vi "Excel_Insert_Table.vi"(0 "worksheet":refnum<k7>, 1 "font":T1 {"font size" format="%0.2f"; "strike through" items=["Unchanged", "Yes", "No"]; "underline" items=["Unchanged", "Yes", "No"]; "italic" items=["Unchanged", "Yes", "No"]; "bold" items=["Unchanged", "Yes", "No"]}, 2 "show grid lines":bool=TRUE, 3 "measurement system":u16(ring) caption="measurement system\nfor column width (US)" items=["US", "Metric"], 5 "column width (1)":dbl=-1.0 format="%0.2f", 7 "table":string[][](table), 11 "error in (no error)":errorcluster, 12 "Start row":i32, 13 "Start column":i32, 14 "name":string) -> (8 "Row":i32, 10 "Column":i32, 15 "error out":errorcluster)   [LabVIEW 2020, in "NI_ReportGenerationToolkit.lvlib"]
uses:
  <vilib>/addons/_office/NI_ReportGenerationToolkit.lvlib
  <vilib>/addons/_office/_exclsub.llb/font.ctl
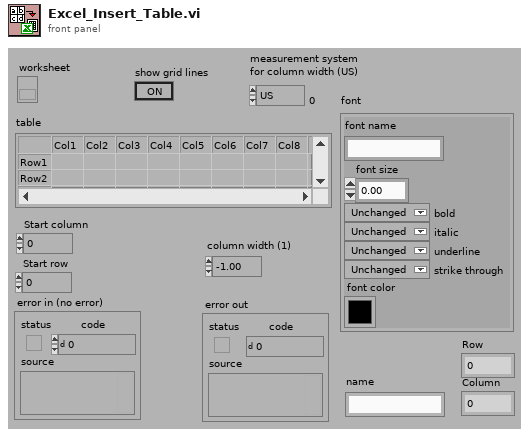
[diagram p1: front panel]
types:
  T1 = typedef "NI_ReportGenerationToolkit.lvlib/font.ctl" = cluster{"font name":string, "font size":dbl, "bold":u16, "italic":u16, "underline":u16, "strike through":u16, "font color":u32}
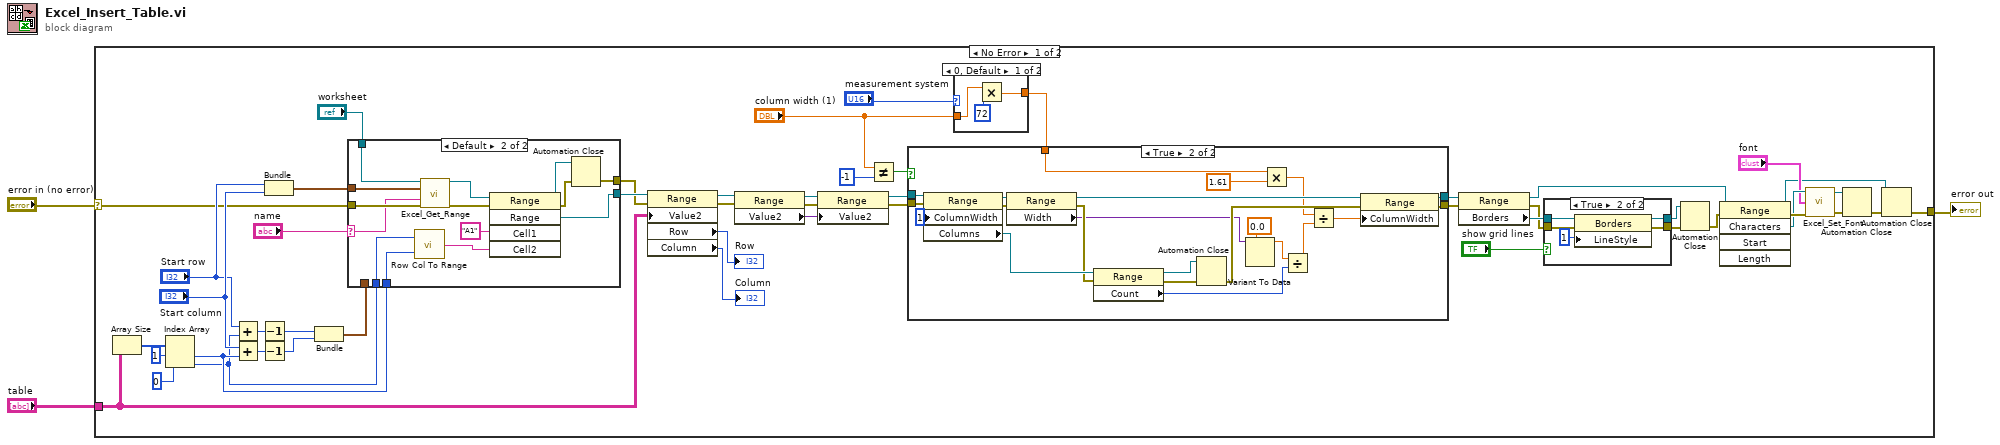
[diagram p0: block diagram]
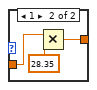
[diagram p2: hidden frame]
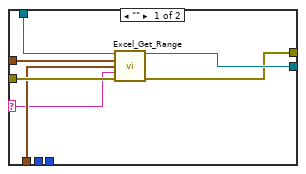
[diagram p4: hidden frame]
diagram:
  n1 = case shown="No Error" "error in (no error)" {
    selector: "error in (no error)" -> [w5 w112]
    tunnel: "table" -> [w44 _]
    tunnel: [w26 w112] -> w2
    frame No Error {
      n2 = Array Size(array=w44) -> (size(s)=w52:i32[])
      n3 = Index Array(array=w52, index #1=1, index #2=0) -> (element #1=w43:i32, element #2=w6:i32)
      n4 = Add(x="Start row", y=w6) -> (x+y=w14:i32)
      n5 = Add(x="Start column", y=w43) -> (x+y=w13:i32)
      n6 = Decrement(x=w14) -> (x-1=w9:i32)
      n7 = Decrement(x=w13) -> (x-1=w8:i32)
      n8 = Bundle("Start row"="Start row", "Start column"="Start column") -> (w15:cluster{"Start row":i32, "Start column":i32})  [unwired: 1 out]
      n9 = Bundle(w9, w8) -> (w12:cluster{i32, i32})  [unwired: 1 out]
      n10 = case shown="Default" "name" {
        selector: "name" -> [w84 w92]
        tunnel: [w90 w104] -> w51
        tunnel: [w89 w98] -> w50
        tunnel: "worksheet" -> [w88 w95]
        tunnel: w5 -> [w87 w94]
        tunnel: w6 -> [_ w100]
        tunnel: w43 -> [_ w101]
        tunnel: w15 -> [w86 w93]
        tunnel: w12 -> [w85 _]
        frame "" {
          n11 = call <vilib>:"Excel_Get_Range.vi"("Excel._Worksheet"=w88, "start"=w86, "end"=w85, "name"=w84, "error in (no error)"=w87) -> ("Range"=w90:refnum<k7>, "error out"=w89:errorcluster)  [unwired: 1 in, 8 out]
        }
        frame Default {
          n12 = call <vilib>:"Row Col To Range.vi"("Column"=w101, "Row"=w100) -> ("Output String"=w102:string)
          n13 = call <vilib>:"Excel_Get_Range.vi"("Excel._Worksheet"=w95, "start"=w93, "name"=w92, "error in (no error)"=w94) -> ("Range"=w91:refnum<k7>, "error out"=w96:errorcluster)  [unwired: 1 in, 9 out]
          n14 = invoke class="Range" method="Range"(reference=w91, error in=w96, "Cell1"="A1", "Cell2"=w102) -> (reference out=w97:refnum<k7>, error out=w99:errorcluster, "Range"=w104:refnum<k7>)  [unwired: 1 in, 2 out]
          n15 = Automation Close(3:w99, 5:w97) -> (0:w98:errorcluster)
        }
      }
      n16 = property class="Range"(reference=w51, error in=w50, "Value2"=w44) -> (reference out=w20:refnum<k7>, error out=w19:errorcluster, "Row"=→"Row":i32, "Column"=→"Column":i32)
      n17 = property class="Range"(reference=w20, error in=w19) -> (reference out=w22:refnum<k7>, error out=w21:errorcluster, "Value2"=w16:variant)
      n18 = property class="Range"(reference=w22, error in=w21, "Value2"=w16) -> (reference out=w18:refnum<k7>, error out=w17:errorcluster)
      n19 = Not Equal?(x="column width (1)", y=-1) -> (x != y?=w45:bool)
      n20 = case shown="0, Default" "measurement system" {
        tunnel: "column width (1)" -> [w56 w58]
        tunnel: [w55 w57] -> w41
        frame 0, Default {
          n21 = Multiply(x=w56, y=72) -> (x*y=w55:dbl)
        }
        frame 1 {
          n22 = Multiply(x=w58, y=28.35) -> (x*y=w57:dbl)
        }
      }
      n23 = case shown="True" w45 {
        tunnel: w18 -> [w61 w83]
        tunnel: w17 -> [w60 w82]
        tunnel: [w60 w80] -> w39
        tunnel: [w61 w81] -> w40
        tunnel: w41 -> [_ w62]
        frame False {
        }
        frame True {
          n24 = property class="Range"(reference=w83, error in=w82, "ColumnWidth"=1) -> (reference out=w69:refnum<k7>, error out=w67:errorcluster, "Columns"=w78:refnum<k7>)
          n25 = property class="Range"(reference=w69, error in=w67) -> (reference out=w68:refnum<k7>, error out=w66:errorcluster, "Width"=w65:variant)
          n26 = property class="Range"(reference=w78, error in=w66) -> (reference out=w74:refnum<k7>, error out=w73:errorcluster, "Count"=w76:i32)
          n27 = Automation Close(3:w73, 5:w74) -> (0:w72:errorcluster)
          n28 = Variant To Data(type=0.0, Variant=w65) -> (data=w77:dbl)  [unwired: 1 in, 1 out]
          n29 = Multiply(x=w62, y=1.61) -> (x*y=w64:dbl)
          n30 = Divide(x=w77, y=w76) -> (x/y=w75:dbl)
          n31 = Divide(x=w64, y=w75) -> (x/y=w71:dbl)
          n32 = property class="Range"(reference=w68, error in=w72, "ColumnWidth"=w71) -> (reference out=w81:refnum<k7>, error out=w80:errorcluster)
        }
      }
      n33 = property class="Range"(reference=w40, error in=w39) -> (reference out=w36:refnum<k7>, error out=w37:errorcluster, "Borders"=w38:refnum<k7>)
      n34 = case shown="True" "show grid lines" {
        tunnel: w38 -> [w105 w110]
        tunnel: w37 -> [w106 w109]
        tunnel: [w106 w108] -> w35
        tunnel: [w105 w107] -> w34
        frame False {
        }
        frame True {
          n35 = property class="Borders"(reference=w110, error in=w109, "LineStyle"=1) -> (reference out=w107:refnum<k7>, error out=w108:errorcluster)
        }
      }
      n36 = Automation Close(3:w35, 5:w34) -> (0:w33:errorcluster)
      n37 = invoke class="Range" method="Characters"(reference=w36, error in=w33) -> (reference out=w27:refnum<k7>, error out=w32:errorcluster, "Characters"=w30:refnum<k7>)  [unwired: 3 in, 2 out]
      n38 = call <vilib>:"Excel_Set_Font.vi"("Excel.Characters"=w30, "font"="font", "error in (no error)"=w32) -> ("Excel.Characters out"=w28:refnum<k7>, "error out"=w31:errorcluster)  [unwired: 5 out]
      n39 = Automation Close(3:w31, 5:w28) -> (0:w49:errorcluster)
      n40 = Automation Close(3:w49, 5:w27) -> (0:w26:errorcluster)
    }
    frame Error {
    }
  }
  "error out" <- w2
